vi "WriteTCPIP.vi"(3 "error in":errorcluster, 4 "String":string, 5 "connection ID":refnum<k5>) -> (0 "errorout":errorcluster, 2 "connection ID Out":refnum<k5>)   [LabVIEW 2012]
panel:
  out "bytes written":i32
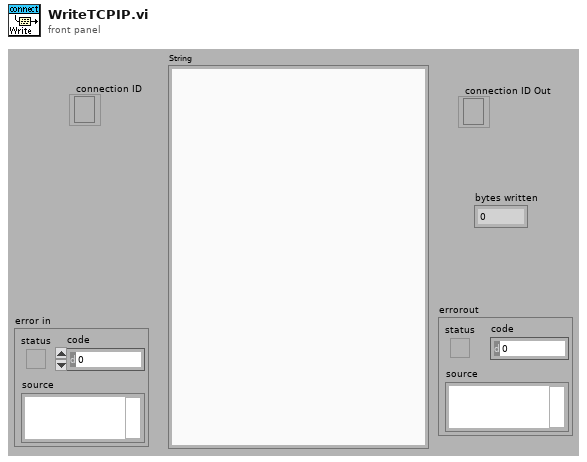
[diagram p1: front panel]
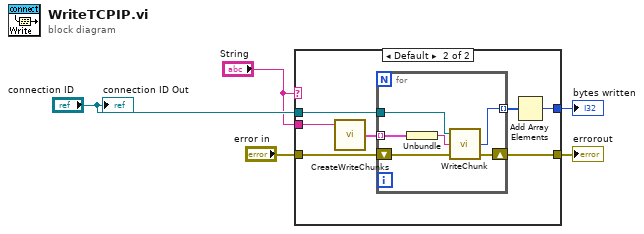
[diagram p0: block diagram]
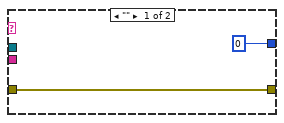
[diagram p2: hidden frame]
diagram:
  n1 = case shown="Default" "String" {
    tunnel: "String" -> [_ w10]
    tunnel: [0 ("bytes written") w8] -> w5
    tunnel: [w7 w11] -> w4
    tunnel: "error in" -> [w7 w12]
    tunnel: "connection ID" -> [_ w14]
    frame "" {
    }
    frame Default {
      n2 = call <userlib>:"CreateWriteChunks.vi"("String"=w10) -> ("chuncks"=w9:cluster{"result string":string}[])  [unwired: 2 in]
      n3 = for {
        tunnel: w14 -> [w20]
        tunnel: [w19] -> w13 mode=indexing
        shift-right: [w17] -> w11
        shift-left: w12 -> [w18]
        tunnel: w9 -> [w16] mode=indexing
        n4 = Unbundle(w16) -> ("result string"=w15:string)
        n5 = call <userlib>:"WriteChunk.vi"("error in (no error)"=w18, "data in"=w15, "connection ID"=w20) -> ("error out"=w17:errorcluster, "bytes written"=w19:i32)  [unwired: 1 out]
      }
      n6 = Add Array Elements(numeric array=w13) -> (sum=w8:i32)
    }
  }
  "errorout" <- w4
  "bytes written" <- w5
  "connection ID Out" <- "connection ID"
